vi "Assert Not Error Code.vi"(4 "Execution time (s)":dbl=-1.0, 5 "Assert Only? (F)":bool, 6 "error code (1)":i32=1, 7 "Label (\"\")":string, 8 "error in (no error)":errorcluster, 9 "Register with caller test (F)":bool, 10 "Error Code":i32, 11 "Error?":errorcluster) -> (0 "error out":errorcluster, 2 "Properties.Assert":refnum<class "Properties.Assert.lvclass">)   [LabVIEW 2013, in "Caraya.lvlib" / "Assert.lvclass"]
doc: "Asserts that <B>Error?</B> is not an error with the specified <B>Error Code</B>."
uses:
  Assert.lvclass
  Properties.Assert/Properties.Assert.lvclass
  Properties/Properties.lvclass
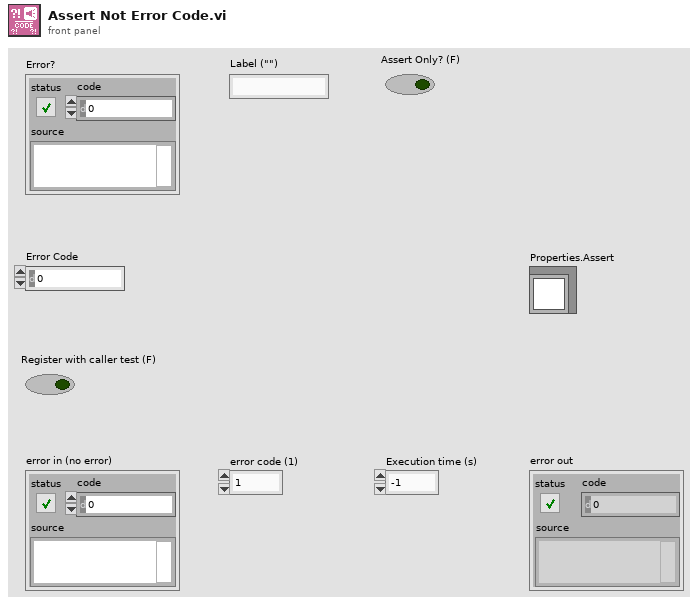
[diagram p1: front panel]
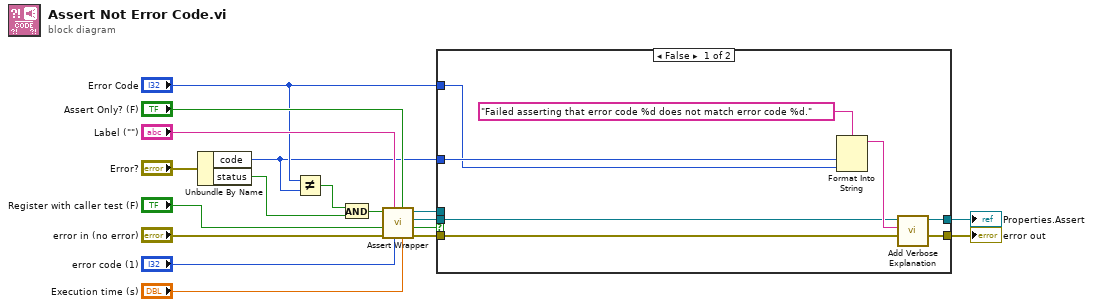
[diagram p0: block diagram]
diagram:
  n1 = Unbundle By Name("Error?") -> ("code"=w4:i32, "status"=w1:bool)
  n2 = Not Equal?(x="Error Code", y=w4) -> (x != y?=w2:bool)
  n3 = And(x=w2, y=w1) -> (x .and. y?=w3:bool)
  n4 = call "Assert Wrapper.vi"("Execution time (s)"="Execution time (s)", "Assert Only? (F)"="Assert Only? (F)", "error code (1)"="error code (1)", "Label"="Label (\"\")", "error in (no error)"="error in (no error)", "Register with caller test (F)"="Register with caller test (F)", "Assert?"=w3) -> ("error out"=w7:errorcluster, "Verbose"=w11:bool, "Properties.Assert"=w9:refnum<class "Properties.Assert.lvclass">, "Assert out"=w10:refnum<class "Assert.lvclass">)  [unwired: 1 in]
  n5 = case shown="False" w11 {
    tunnel: w10 -> [_ _]
    tunnel: w9 -> [w21 w28]
    tunnel: [w23 w27] -> w8
    tunnel: w7 -> [w24 w27]
    tunnel: "Error Code" -> [w25 _]
    tunnel: w4 -> [w26 _]
    tunnel: [w20 w28] -> w6
    frame False {
      n6 = Format Into String(format string="Failed asserting that error code %d does not match error code %d.", w26, w25) -> (resulting string=w22:string)  [unwired: 2 in, 1 out]
      n7 = call "Add Verbose Explanation.vi"("error in (no error)"=w24, "Verbose Explanation"=w22, "Properties"=w21) -> ("error out"=w23:errorcluster, "Properties"=w20:refnum<class "Properties.Assert.lvclass">)  [unwired: 7 in]
    }
    frame True {
    }
  }
  "error out" <- w8
  "Properties.Assert" <- w6
